vi "ReadConfiguration.vi"(8 "Error In":errorcluster, 11 "VI Path":path) -> (0 "Error Out":errorcluster, 3 "Executable Configuration":T1)   [LabVIEW 2012]
uses:
  ExecutableConfiguration.ctl
  <vilib>/Utility/config.llb/Read Key (I32).vi
  <vilib>/Utility/config.llb/Read Key (Boolean).vi
  <vilib>/Utility/config.llb/Read Key (String).vi
  <vilib>/Utility/config.llb/Read Key (Path).vi
  <vilib>/Utility/config.llb/NI_LVConfig.lvlib
  libs/LV-Utilities/LV-Utilities.lvlib
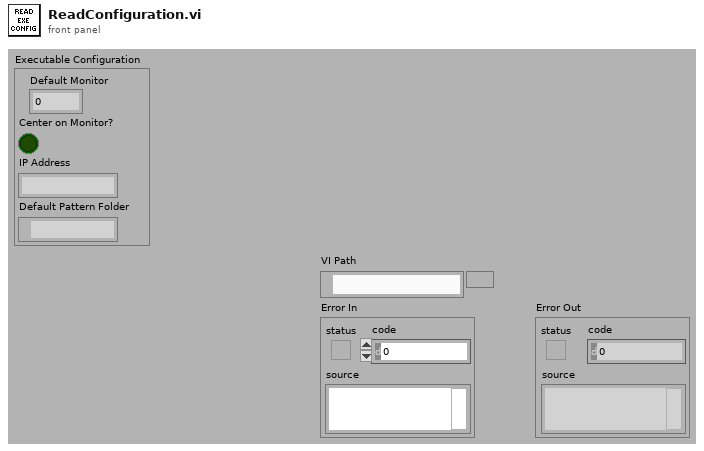
[diagram p1: front panel]
types:
  T1 = typedef "ExecutableConfiguration.ctl" = cluster{"Default Monitor":i32, "Center on Monitor?":bool, "IP Address":string, "Default Pattern Folder":path}
  T2 = typedef "NI_LVConfig.lvlib/Config Data RefNum.ctl" = refnum<k1>
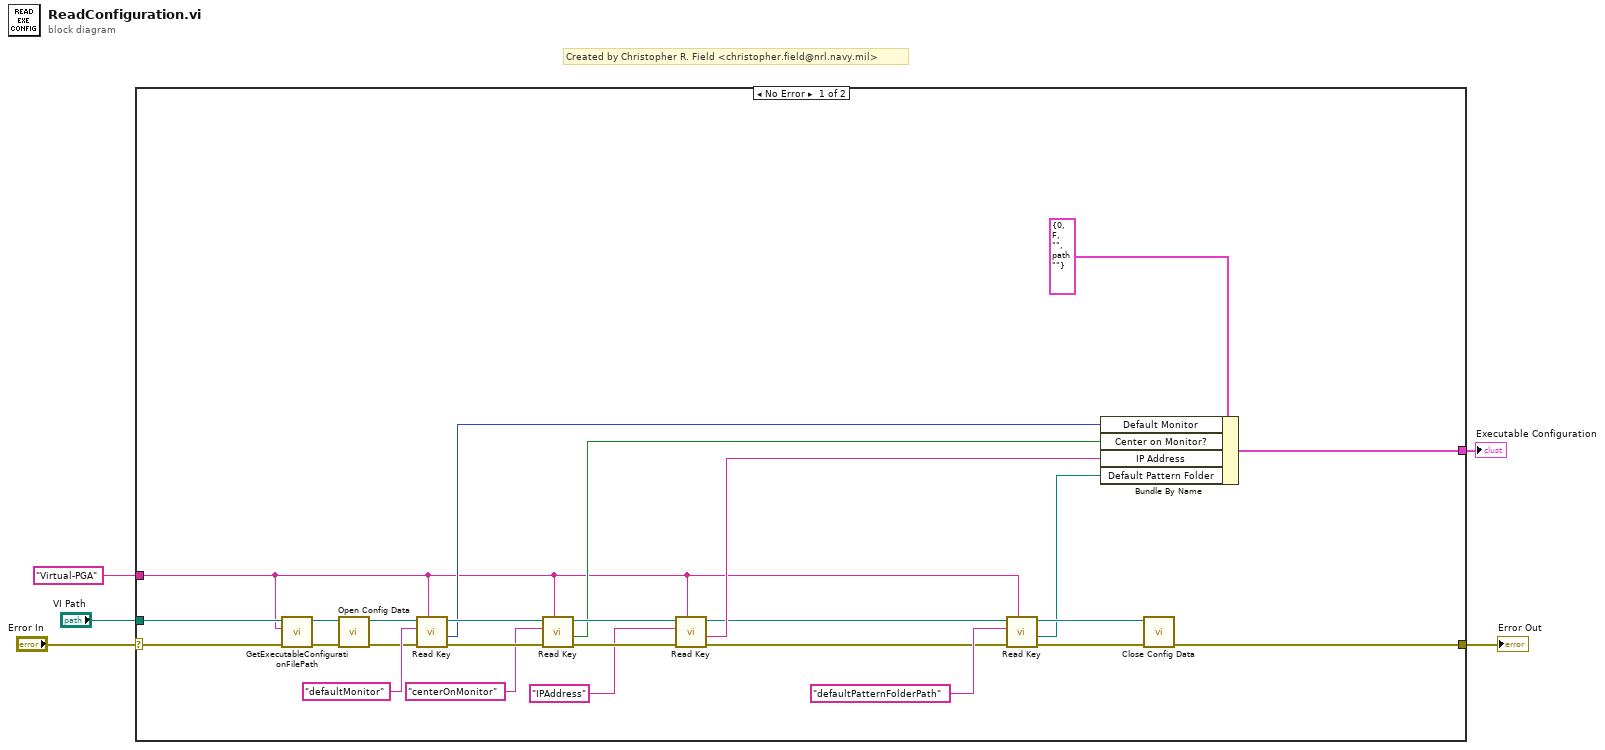
[diagram p0: block diagram]
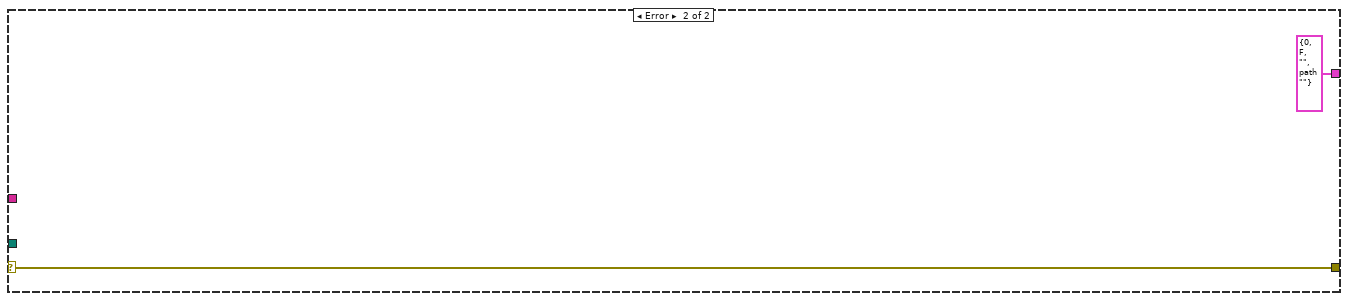
[diagram p2: hidden frame]
diagram:
  # "Created by Christopher R. Field <christopher.field@nrl.navy.mil>"
  n1 = case shown="No Error" "Error In" {
    selector: "Error In" -> [w26 w33]
    tunnel: "VI Path" -> [w25 _]
    tunnel: [w31 w33] -> w4
    tunnel: "Virtual-PGA" ("section") -> [w8 _]
    tunnel: [w9 T1 {"Default Monitor"=0, "Center on Monitor?"=FALSE, "IP Address"="", "Default Pattern Folder"=path ""} ("Executable Configuration")] -> w1
    frame No Error {
      n2 = call "GetExecutableConfigurationFilePath.vi"("Error In"=w26, "Application Name"=w8, "VI Path"=w25) -> ("Error Out"=w23:errorcluster, "Executable Config File Path"=w24:path)  [unwired: 7 in]
      n3 = call <vilib>:"Open Config Data.vi"("error in (no error)"=w23, "configuration file path"=w24) -> ("error out"=w21:errorcluster, "refnum"=w22:T2)  [unwired: 7 in, 1 out]
      n4 = call-poly <vilib>:"Read Key.vi"("section"=w8, "error in (no error)"=w21, "key"="defaultMonitor", "refnum"=w22) -> ("error out"=w19:errorcluster, "value"=w13:i32, "refnum out"=w20:T2)  [unwired: 4 in, 1 out]
      n5 = call-poly <vilib>:"Read Key.vi"("section"=w8, "error in (no error)"=w19, "key"="centerOnMonitor", "refnum"=w20) -> ("error out"=w16:errorcluster, "value"=w12:bool, "refnum out"=w17:T2)  [unwired: 4 in, 1 out]
      n6 = call-poly <vilib>:"Read Key.vi"("section"=w8, "error in (no error)"=w16, "key"="IPAddress", "refnum"=w17) -> ("error out"=w6:errorcluster, "value"=w11:string, "refnum out"=w7:T2)  [unwired: 4 in, 1 out]
      n7 = call-poly <vilib>:"Read Key.vi"("section"=w8, "error in (no error)"=w6, "key"="defaultPatternFolderPath", "refnum"=w7) -> ("error out"=w28:errorcluster, "value"=w10:path, "refnum out"=w29:T2)  [unwired: 4 in, 1 out]
      n8 = Bundle By Name(cluster=T1 {"Default Monitor"=0, "Center on Monitor?"=FALSE, "IP Address"="", "Default Pattern Folder"=path ""} ("Executable Configuration"), "Default Monitor"=w13, "Center on Monitor?"=w12, "IP Address"=w11, "Default Pattern Folder"=w10) -> (w9:T1)
      n9 = call <vilib>:"Close Config Data.vi"("error in (no error)"=w28, "refnum"=w29) -> ("error out"=w31:errorcluster)  [unwired: 8 in, 1 out]
    }
    frame Error {
    }
  }
  "Error Out" <- w4
  "Executable Configuration" <- w1
